vi "ief_close_connections.vi"(2 "error in (no error)":errorcluster, 3 "Tagprefix in":refnum<k21>) -> (0 "error out (no error)":errorcluster, 1 "Tagprefix out":refnum<k21>)   [LabVIEW 2015, in "IEF Werner.lvlib"]
doc: "Closes the SV connection to all necessary variables."
uses:
  IEF Werner.lvlib
  Packages/CSPP_Core/Libraries/Base/FGV Action.ctl
  Packages/CSPP_Core/Libraries/Base/CS++Base.lvlib
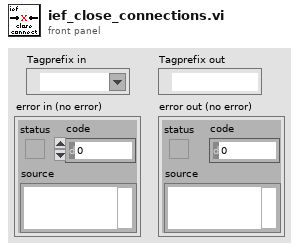
[diagram p1: front panel]
types:
  T1 = typedef "CS++Base.lvlib/FGV Action.ctl" = enum16{"add", "replace", "read", "remove", "reset", "get attributes"}
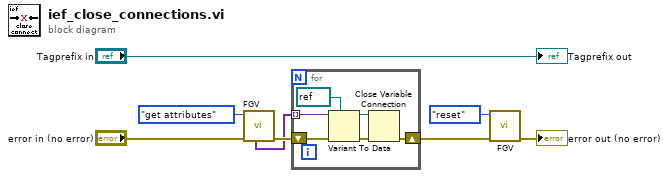
[diagram p0: block diagram]
diagram:
  n1 = call "FGV.vi"("Error In"="error in (no error)", "Action (read)"=FGV_Action."get attributes") -> ("Error Out"=w5:errorcluster, "Attribute Values"=w4:variant[])  [unwired: 5 in, 3 out]
  n2 = for {
    tunnel: w4 -> [w14] mode=indexing
    shift-right: [w11] -> w3
    shift-left: w5 -> [w13]
    n3 = Variant To Data(error in=w13, type=refnum<k21> refnum ("shared variable refnum in"), Variant=w14) -> (data=w9:refnum<k21>, error out=w12:errorcluster)
    n4 = Close Variable Connection(8:w12, 11:w9) -> (0:w11:errorcluster)
  }
  n5 = call "FGV.vi"("Error In"=w3, "Action (read)"=FGV_Action."reset") -> ("Error Out"=→"error out (no error)":errorcluster)  [unwired: 5 in, 4 out]
  "Tagprefix out" <- "Tagprefix in"
